vi "Lpeak.vi"(11 "Numeric":dbl) -> (3 "Lpeak":dbl)   [LabVIEW 2020]
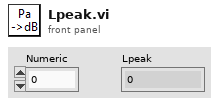
[diagram p1: front panel]
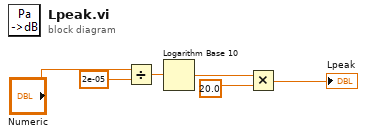
[diagram p0: block diagram]
diagram:
  n1 = Divide(x="Numeric", y=2e-05) -> (x/y=w1:dbl)
  n2 = Logarithm Base 10(1:w1) -> (0:w2:dbl)
  n3 = Multiply(x=w2, y=20.0) -> (x*y=→"Lpeak":dbl)
